vi "Create Table Range.vi"(8 "error in":errorcluster, 9 "Range or Cell Address":string, 10 "Header Names":string[](array[string]), 11 "Values":variant[][](array[variant])) -> (0 "error out":errorcluster, 3 "Table Range":string)   [LabVIEW 2019, in "Open Xml.lvlib"]
uses:
  Open Xml.lvlib
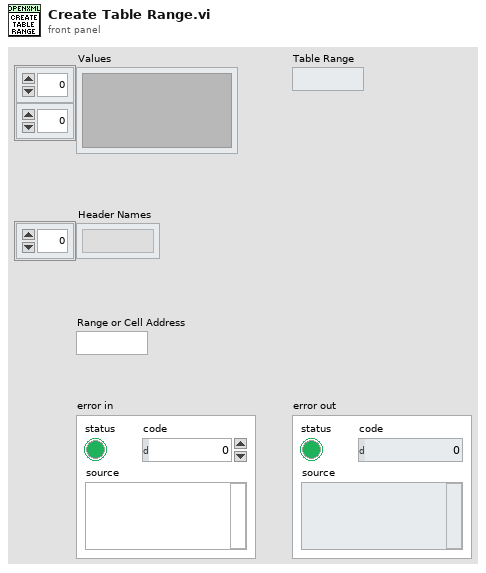
[diagram p1: front panel]
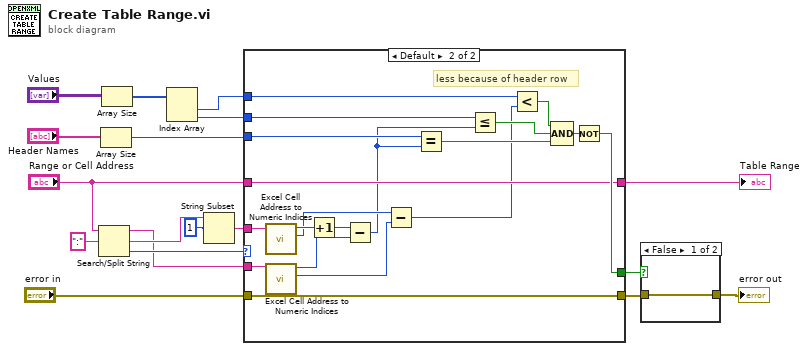
[diagram p0: block diagram]
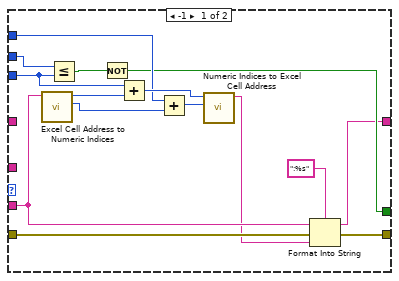
[diagram p2: hidden frame]
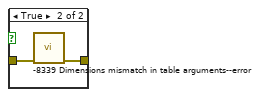
[diagram p3: hidden frame]
diagram:
  n1 = Search/Split String(string="Range or Cell Address", search string/char (-)=":") -> (substring before match=w11:string, match + rest of string=w14:string, offset of match=w15:i32)  [unwired: 1 in]
  n2 = Array Size(array="Header Names") -> (size(s)=w10:i32)
  n3 = Array Size(array="Values") -> (size(s)=w9:i32[])
  n4 = Index Array(array=w9) -> (element #1=w8:i32, element #2=w7:i32)  [unwired: 2 in]
  n5 = String Subset(string=w14, offset (0)=1) -> (substring=w12:string)  [unwired: 1 in]
  n6 = case shown="Default" w15 {
    tunnel: w12 -> [_ w52]
    tunnel: w11 -> [w22 w51]
    tunnel: w10 -> [w31 w50]
    tunnel: w8 -> [w29 w48]
    tunnel: w7 -> [w32 w49]
    tunnel: "error in" -> [w24 w44]
    tunnel: [w23 w44] -> w4
    tunnel: [w25 w42] -> w3
    tunnel: [w19 w41] -> w2
    tunnel: "Range or Cell Address" -> [_ w41]
    frame -1 {
      n7 = call "Excel Cell Address to Numeric Indices.vi"("Cell Name"=w22) -> ("Row Number"=w28:i32, "Column Number"=w33:i32)  [unwired: 9 in]
      n8 = Less Or Equal?(x=w32, y=w31) -> (x <= y?=w26:bool)
      n9 = Not(x=w26) -> (.not. x?=w25:bool)
      n10 = Add(x=w31, y=w33) -> (x+y=w30:i32)
      n11 = Add(x=w29, y=w28) -> (x+y=w27:i32)
      n12 = call "Numeric Indices to Excel Cell Address.vi"("Row"=w27, "Column"=w30) -> ("Cell Address"=w20:string)  [unwired: 9 in]
      n13 = Format Into String(format string=":%s", initial string=w22, error in=w24, w20) -> (resulting string=w19:string, error out=w23:errorcluster)
    }
    frame Default {
      # "less because of header row"
      n14 = call "Excel Cell Address to Numeric Indices.vi"("Cell Name"=w52) -> ("Row Number"=w36:i32, "Column Number"=w40:i32)  [unwired: 9 in]
      n15 = call "Excel Cell Address to Numeric Indices.vi"("Cell Name"=w51) -> ("Row Number"=w37:i32, "Column Number"=w39:i32)  [unwired: 9 in]
      n16 = Increment(x=w40) -> (x+1=w35:i32)
      n17 = Subtract(x=w35, y=w39) -> (x-y=w34:i32)
      n18 = Subtract(x=w36, y=w37) -> (x-y=w38:i32)
      n19 = Equal?(x=w50, y=w34) -> (x = y?=w45:bool)
      n20 = Less Or Equal?(x=w49, y=w34) -> (x <= y?=w46:bool)
      n21 = Less?(x=w48, y=w38) -> (x < y?=w47:bool)
      n22 = Compound Arithmetic op=AND(w47, w46, w45) -> (w43:bool)
      n23 = Not(x=w43) -> (.not. x?=w42:bool)
    }
  }
  "Table Range" <- w2
  n24 = case shown="False" w3 {
    tunnel: w4 -> [w53 w55]
    tunnel: [w53 w54] -> w5
    frame False {
    }
    frame True {
      n25 = call "-8339 Dimensions mismatch in table arguments--error.vi"("error in"=w55) -> ("error out"=w54:errorcluster)  [unwired: 9 in, 1 out]
    }
  }
  "error out" <- w5
